vi "Rcv Cmd.vi"(8 "error in":errorcluster, 11 "nCRD in":refnum<class "nCRD.lvclass">) -> (0 "error out":errorcluster, 3 "nCRD out":refnum<class "nCRD.lvclass">)   [LabVIEW 2014, in "nCRD.lvclass"]
uses:
  nCRD.lvclass
  Reusable/Instrument/state.ctl
  Reusable/Instrument/Instrument.lvclass
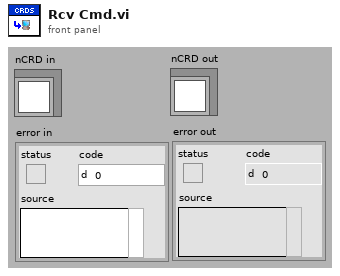
[diagram p1: front panel]
types:
  T1 = typedef "Instrument.lvclass/state.ctl" = enum8{"Configure", "Acquire", "Wait", "Quit", "Handle Error", "NOOP"}
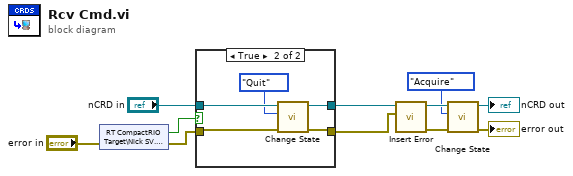
[diagram p0: block diagram]
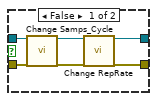
[diagram p2: hidden frame]
diagram:
  n1 = shared-variable "RT CompactRIO Target\\Nick SV.lvlib\\Stop"(error in="error in") -> (w11:bool, error out=w9:errorcluster)
  n2 = case shown="True" w11 {
    tunnel: w9 -> [w12 w20]
    tunnel: "nCRD in" -> [w13 w22]
    tunnel: [w15 w19] -> w5
    tunnel: [w14 w18] -> w4
    frame False {
      n3 = call "Change Samps_Cycle.vi"("nCRD in"=w13, "error in"=w12) -> ("nCRD out"=w16:refnum<class "nCRD.lvclass">, "error out"=w17:errorcluster)  [unwired: 16 in]
      n4 = call "Change RepRate.vi"("nCRD in"=w16, "error in"=w17) -> ("nCRD out"=w15:refnum<class "nCRD.lvclass">, "error out"=w14:errorcluster)  [unwired: 16 in]
    }
    frame True {
      n5 = call "Change State.vi"("error in"=w20, "instr state"=state."Quit", "Instrument in"=w22) -> ("error out"=w18:errorcluster, "Instrument out"=w19:refnum<class "nCRD.lvclass">)  [unwired: 7 in]
    }
  }
  n6 = call "Insert Error.vi"("err"=w4, "Instrument in"=w5) -> ("error out"=w1:errorcluster, "Instrument out"=w3:refnum<class "nCRD.lvclass">)  [unwired: 7 in, 1 out]
  n7 = call "Change State.vi"("error in"=w1, "instr state"=state."Acquire", "Instrument in"=w3) -> ("error out"=→"error out":errorcluster, "Instrument out"=→"nCRD out":refnum<class "nCRD.lvclass">)  [unwired: 7 in]
